vi "parse.vi"(8 "error in (no error)":errorcluster, 9 "SwapBytes":bool, 10 "Data":u8[](array[numeric]), 11 "U8ArrayParserAutoIndexing in":refnum<class "U8ArrayParserAutoIndexing.lvclass">) -> (0 "error out":errorcluster, 3 "U8ArrayParserAutoIndexing out":refnum<class "U8ArrayParserAutoIndexing.lvclass">)   [LabVIEW 2016, in "RTUtilities.lvlib" / "U8ArrayParserAutoIndexing.lvclass"]
uses:
  U8ArrayParserAutoIndexing.lvclass
  U8ArrayParser/U8ArrayParserManualIndexing.lvclass
  U8ArrayParserAutoIndexing.lvclass/U8ArrayParserAutoIndexing.ctl
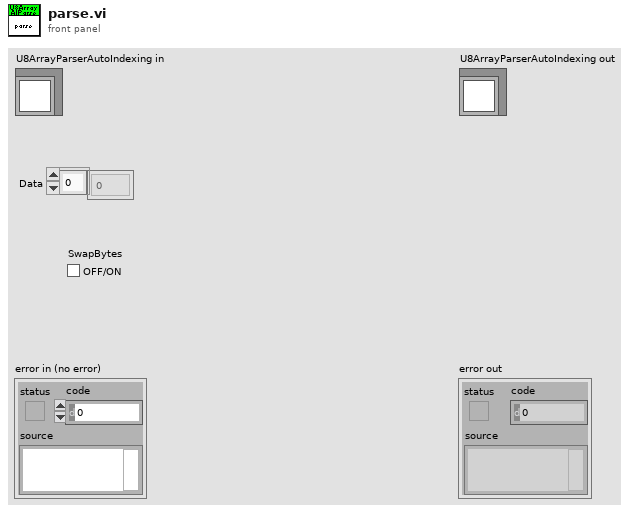
[diagram p1: front panel]
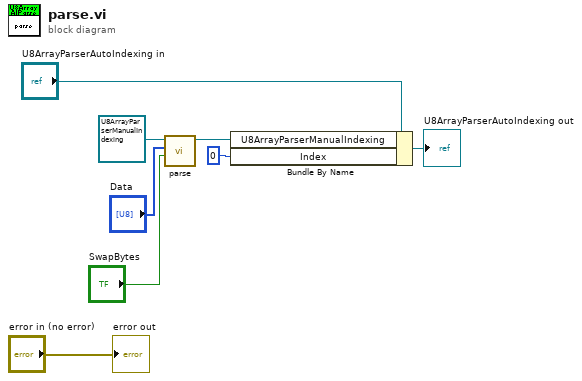
[diagram p0: block diagram]
diagram:
  n1 = call "parse.vi"("SwapBytes"="SwapBytes", "Data"="Data", "U8ArrayParserManualIndexing in"=refnum<class "U8ArrayParserManualIndexing.lvclass"> refnum ("RTUtilities.lvlib:U8ArrayParserManualIndexing.lvclass")) -> ("U8ArrayParserManualIndexing out"=w2:refnum<class "U8ArrayParserManualIndexing.lvclass">)  [unwired: 7 in, 1 out]
  n2 = Bundle By Name(cluster="U8ArrayParserAutoIndexing in", "U8ArrayParserManualIndexing"=w2, "Index"=0) -> (→"U8ArrayParserAutoIndexing out":refnum<class "U8ArrayParserAutoIndexing.lvclass">)
  "error out" <- "error in (no error)"
